vi "ReadMutationHistoryPathWrapper.vi"(8 "error in (no error)":errorcluster, 9 "Name":string, 10 "LVClass path":path, 11 "Application":refnum<vi>) -> (0 "error out":errorcluster, 3 "Application":refnum<vi>)   [LabVIEW 2019, in "BlueSerializationScripts.lvlib"]
uses:
  BlueSerializationScripts.lvlib
  UserAppLibs/MutationHistoryGUI/MutationHistoryGUI.lvlib
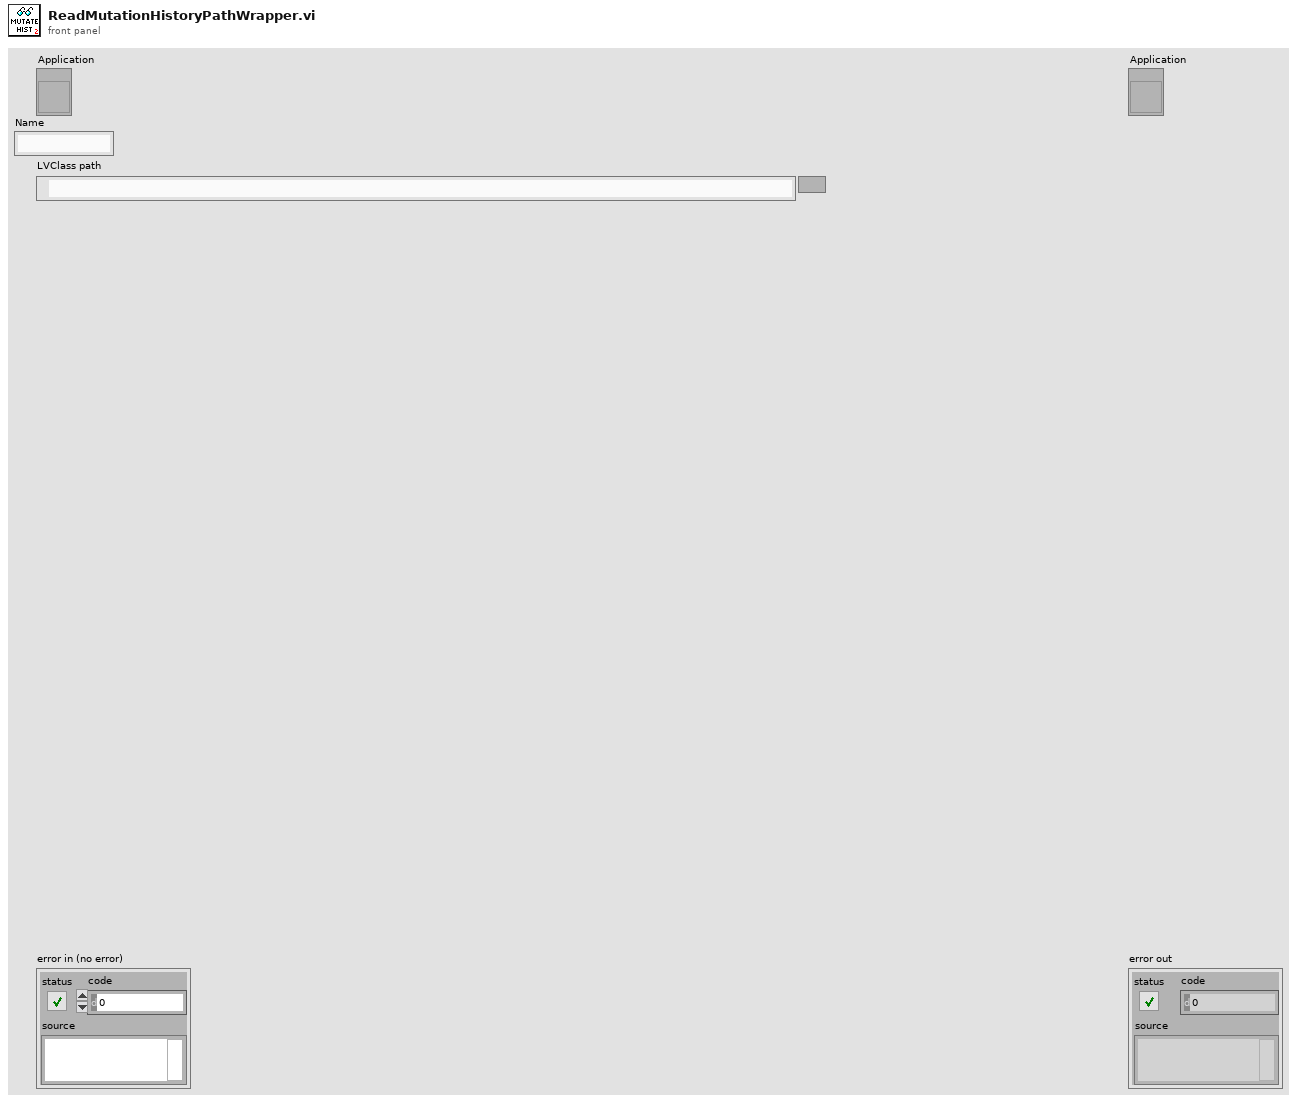
[diagram p1: front panel]
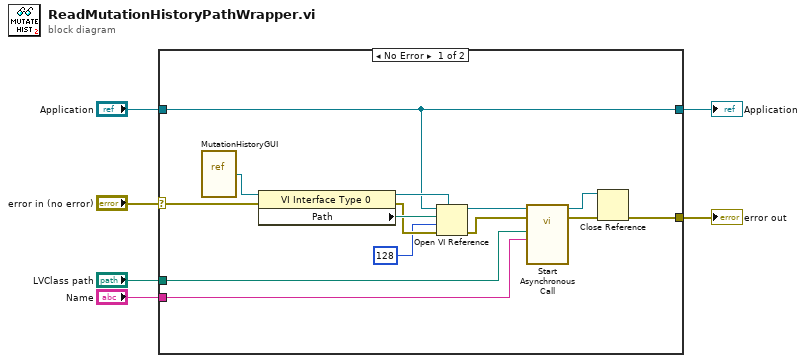
[diagram p0: block diagram]
diagram:
  n1 = case shown="No Error" "error in (no error)" {
    selector: "error in (no error)" -> [w12 w22]
    tunnel: [w8 w22] -> w6
    tunnel: [w11 w21] -> w5
    tunnel: "LVClass path" -> [w10 _]
    tunnel: "Application" -> [w11 w21]
    tunnel: "Name" -> [w9 _]
    frame No Error {
      n2 = vi-ref "MutationHistoryGUI.vi"() -> (w20:refnum<vi>)
      n3 = property class="VI Interface Type 0"(reference=w20, error in=w12) -> (reference out=w18:refnum<vi>, error out=w17:errorcluster, "Path"=w19:path)
      n4 = Open VI Reference(type specifier VI Refnum (for type only)=w18, application reference (local)=w11, vi path=w19, options=128, error in (no error)=w17) -> (vi reference=w16:refnum<vi>, error out=w15:errorcluster)  [unwired: 1 in]
      n5 = call-by-ref "Start Asynchronous Call"(reference=w16, error in=w15, "Title"=w9, "LVClass path"=w10) -> (reference out=w14:refnum<vi>, error out=w13:errorcluster)  [unwired: 10 in]
      n6 = Close Reference(reference=w14, error in (no error)=w13) -> (error out=w8:errorcluster)
    }
    frame Error {
    }
  }
  "error out" <- w6
  "Application" <- w5
